vi "CreateListener.vi"(8 "error in (no error)":errorcluster, 11 "qbus":refnum<class "Qbus.lvclass">) -> (0 "error out":errorcluster, 3 "qbus out":refnum<class "Qbus.lvclass">)   [LabVIEW 2017, in "CmsAcquisition.lvlib"]
uses:
  <vilib>/addons/InsightCM/Devices/Shared/Cms/CmsAcquisition/CmsAcquisition.lvlib
  <vilib>/addons/Qbus/Qbus.lvclass
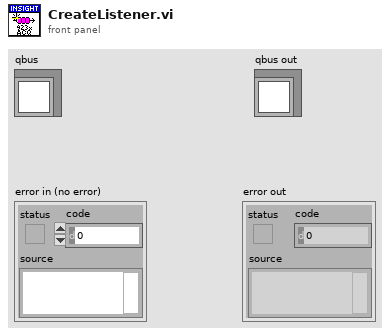
[diagram p1: front panel]
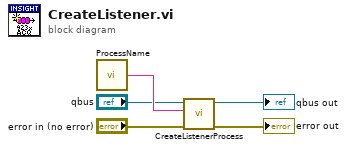
[diagram p0: block diagram]
diagram:
  n1 = call <vilib>:"ProcessName.vi"() -> ("process name"=w5:string)  [unwired: 5 in]
  n2 = call <vilib>:"CreateListenerProcess.vi"("error in (no error)"="error in (no error)", "process name"=w5, "Qbus in"="qbus") -> ("error in (no error)"=→"error out":errorcluster, "Qbus out"=→"qbus out":refnum<class "Qbus.lvclass">)  [unwired: 7 in]
